vi "数据库.vi"() -> ()   [LabVIEW 2020]
panel:
  in  "db file":path
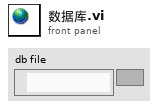
[diagram p1: front panel]
diagram:
